vi "DUT Power Sequence.vi"(0 "TSM context":T2, 1 "SMU Current Limit (A)":dbl=0.01 format="%#_6p", 5 "Power Sequence":T1[](array[typedef]) {"Delay after Set" format="%#_6p"; "Level (V)" format="%#_6p"}, 12 "PPMU Current Limit  Range (A)":dbl=0.01 format="%#_6p") -> (15 "error out":errorcluster)   [LabVIEW 2020]
doc: "Use this VI to power up a DUT using NI SMU(s) with the NI-DCPower driver or digital PPMU(s) with the NI-Digital Pattern Driver. You can provide input values to the step to specify the voltage and current to use to power up the DUT.\n\nThe DUT Power Up VI also measures the voltage and current of each pin once the power up operation is complete. Configure test evaluations on the Tests tab of the Step Settings pane in TestStand to evaluate the results of these measurements."
uses:
  <vilib>/NI_TestStand_SemiconductorModule/NI_TestStand_Semiconductor_Module.lvlibp/PinMap/General/SemiconductorModuleContext.ctl
  SubVIs/DUT Power Sequence Example [SW Timed] - Power Sequence Element.ctl
  <vilib>/NI_TestStand_SemiconductorModule/NI_TestStand_Semiconductor_Module.lvlibp/PinMap/General/NIInstrumentTypeIDs.ctl
  23f3df9e-2b2d-485b-a485-3ec9bf7aef5a.vi
  23f3df9e-2b2d-485b-a485-3ec9bf7aef5a.vi/3e263204-4090-4715-a571-9ccab41da9b7.vi
  23f3df9e-2b2d-485b-a485-3ec9bf7aef5a.vi/e8aa53f3-4449-4bd6-b84c-856b724761e6.vi
  23f3df9e-2b2d-485b-a485-3ec9bf7aef5a.vi/c9401653-e070-4a50-9511-853cae294189.vi
  23f3df9e-2b2d-485b-a485-3ec9bf7aef5a.vi/b509eb7d-d7fc-447a-a129-4a3f0498ddd1.vi
  Common/Instrument Control/Digital/SSC Digital/PPMU/SSC Digital PPMU Source Voltage.vi
  Common/Instrument Control/DCPower/SSC DCPower/Source/Constant Voltage/SSC DCPower Force Voltage Array Symmetric Limits.vi
  <vilib>/NI_TestStand_SemiconductorModule/NI_TestStand_Semiconductor_Module.lvlibp
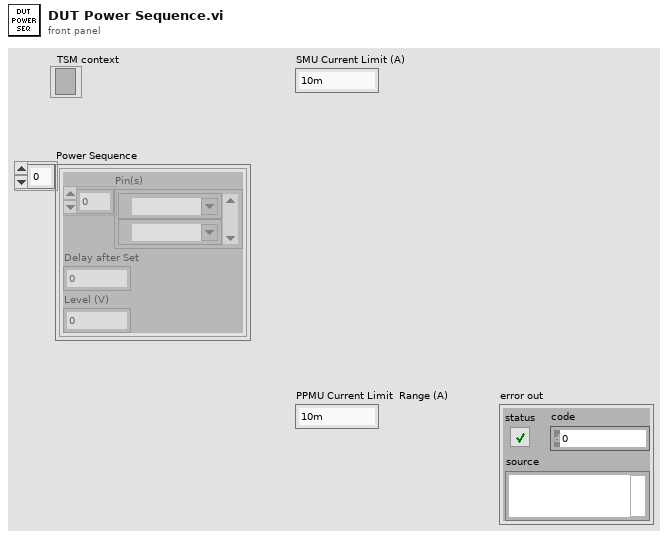
[diagram p1: front panel]
types:
  T1 = typedef "DUT Power Sequence Example [SW Timed] - Power Sequence Element.ctl" = cluster{"Pin(s)":tag[], "Delay after Set":dbl, "Level (V)":dbl}
  T2 = typedef "NI_TestStand_Semiconductor_Module.lvlibp/SemiconductorModuleContext.ctl" = refnum<k7>
  T3 = typedef "NI_TestStand_Semiconductor_Module.lvlibp/NIInstrumentTypeIDs.ctl" = string
  T4 = typedef "NI_TestStand_Semiconductor_Module.lvlibp/TSM_Pin.ctl" = tag
  T5 = typedef "TSM SSC DCPower.ctl" = cluster{"Pin Query Context":refnum<class "MultiplePinMultipleSessionQueryContext.lvclass">, "SSC":T6[], "Site Numbers":i32[], "Pins":T7[], "Pins Expanded":T9[]}
  T6 = typedef "SSC DCPower.ctl" = cluster{"Session":refnum<k15>, "Chan":string, "Channel List":string}
  T7 = typedef "TSM Pin Information.ctl" = cluster{"Pin":tag, "Type":T8, "Count":i32}
  T8 = typedef "TSM Pin Type Identifier.ctl" = enum8{"DUT Pin", "System Pin", "Pin Group", "Not Determined"}
  T9 = typedef "TSM Expanded Pin Information.ctl" = cluster{"Pin":tag, "Type":T8, "Index":i32}
  T10 = typedef "TSM SSC Digital.ctl" = cluster{"Pin Query Context":refnum<class "DigitalPatternPinQueryContext.lvclass">, "SSC":T11[], "Site Numbers":i32[], "Pins":tag[]}
  T11 = typedef "SSC Digital.ctl" = cluster{"Session":refnum<k15>, "Channel List":string, "Site List":string}
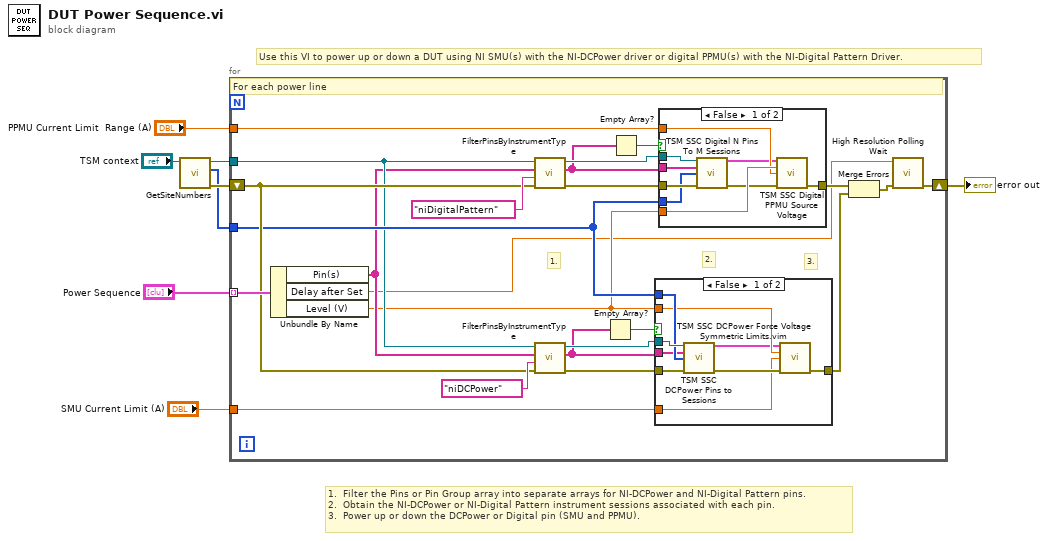
[diagram p0: block diagram]
diagram:
  # "Use this VI to power up or down a DUT using NI SMU(s) with the NI-DCPower driver or digital PPMU(s) with the NI-Digital Pattern Driver."
  # "1.  Filter the Pins or Pin Group array into separate arrays for NI-DCPower and NI-Digital Pattern pins.\n2.  Obtain the NI-DCPower or NI-Digital Pattern instrument sessions associated with each pin.\n3.  Power up or down the DCPower or Digital pin (SMU and PPMU)."
  n1 = call <vilib>:"GetSiteNumbers.vi"("Semiconductor Module Context"="TSM context") -> ("error out"=w5:errorcluster, "Site Numbers"=w4:i32[], "Semiconductor Module Context Out"=w6:T2)  [unwired: 7 in, 1 out]
  n2 = for {
    tunnel: "Power Sequence" -> [w31] mode=indexing
    tunnel: w6 -> [w22]
    shift-right: [w10] -> w1
    shift-left: w5 -> [w24]
    tunnel: w4 -> [w23]
    tunnel: "SMU Current Limit (A)" -> [w19]
    tunnel: "PPMU Current Limit  Range (A)" -> [w18]
    # "3."
    # "2."
    # "1."
    # "For each power line"
    n3 = Unbundle By Name(w31) -> ("Pin(s)"=w21:tag[], "Delay after Set"=w9:dbl, "Level (V)"=w20:dbl)
    n4 = call <vilib>:"FilterPinsByInstrumentType.vi"("error in (no error)"=w24, "Instrument Type Id"=T3 "niDigitalPattern", "Pins"=w21, "Semiconductor Module Context"=w22) -> ("error out"=w27:errorcluster, "Filtered Pins"=w14:T4[], "Semiconductor Module Context Out"=w26:T2)  [unwired: 5 in]
    n5 = call <vilib>:"FilterPinsByInstrumentType.vi"("error in (no error)"=w24, "Instrument Type Id"=T3 "niDCPower", "Pins"=w21, "Semiconductor Module Context"=w22) -> ("error out"=w28:errorcluster, "Filtered Pins"=w13:T4[], "Semiconductor Module Context Out"=w29:T2)  [unwired: 5 in]
    n6 = Empty Array?(array=w13) -> (empty?=w11:bool)
    n7 = Empty Array?(array=w14) -> (empty?=w12:bool)
    n8 = case shown="False" w11 {
      tunnel: w29 -> [w40 _]
      tunnel: w28 -> [w39 w41]
      tunnel: w23 -> [w38 _]
      tunnel: w20 -> [w36 _]
      tunnel: w19 -> [w35 _]
      tunnel: [w34 w41] -> w15
      tunnel: w13 -> [w33 _]
      frame False {
        n9 = call "TSM SSC DCPower Pins to Sessions.vi"("TSM context"=w40, "Pins"=w33, "Site Numbers"=w38, "error in"=w39) -> ("DCPower TSM Out"=w32:T5, "error out"=w37:errorcluster)  [unwired: 10 in]
        n10 = call "TSM SSC DCPower Force Voltage Symmetric Limits.vim"("DCPower TSM in"=w32, "Voltage Level (V)"=w36, "Current Limit (A)"=w35, "error in"=w37) -> ("error out"=w34:errorcluster)  [unwired: 10 in, 1 out]
      }
      frame True {
      }
    }
    n11 = case shown="False" w12 {
      tunnel: w27 -> [w50 w51]
      tunnel: w26 -> [w49 _]
      tunnel: w23 -> [w48 _]
      tunnel: w20 -> [w47 _]
      tunnel: w18 -> [w46 _]
      tunnel: [w42 w51] -> w17
      tunnel: w14 -> [w43 _]
      frame False {
        n12 = call "TSM SSC Digital N Pins To M Sessions.vi"("TSM context"=w49, "Pins"=w43, "Site Numbers"=w48, "error in"=w50) -> ("Digital TSM Out"=w45:T10, "error out"=w44:errorcluster)  [unwired: 10 in]
        n13 = call "TSM SSC Digital PPMU Source Voltage.vi"("Digital TSM In"=w45, "Voltage Level (V)"=w47, "Current Limit Range (A)"=w46, "error in"=w44) -> ("error out"=w42:errorcluster)  [unwired: 10 in, 1 out]
      }
      frame True {
      }
    }
    n14 = Merge Errors(w17, w15) -> (w16:errorcluster)
    n15 = call <vilib>:"High Resolution Polling Wait.vi"("error in (no error)"=w16, "seconds to wait"=w9) -> ("error out"=w10:errorcluster)  [unwired: 9 in]
  }
  "error out" <- w1
